vi "ds get index by serial number.vi"(10 "docking_station_index":u32, 11 "serial_number":u32) -> (2 "docking_station_index out":u32, 3 "function return":i32)   [LabVIEW 2019, in "apdm.lvlib"]
doc: "APDM_EXPORT int apdm_ds_get_index_by_serial_number(const uint32_t serial_number, uint32_t *docking_station_index);"
uses:
  apdm.lvlib
  Lee Lab/CP FES Walking 2018/Code/Working/LabVIEW/apdm.dll
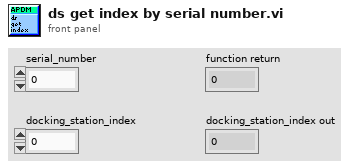
[diagram p1: front panel]
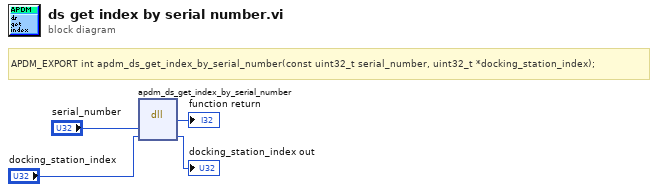
[diagram p0: block diagram]
diagram:
  # "APDM_EXPORT int apdm_ds_get_index_by_serial_number(const uint32_t serial_number, uint32_t *docking_station_index);"
  n1 = dll-call lib="C:/Users/jfalesi/Dropbox/Lee Lab/CP FES Walking 2018/Code/Working/LabVIEW/apdm.*" fn="apdm_ds_get_index_by_serial_number"("serial_number"="serial_number", "docking_station_index"="docking_station_index") -> (→"function return":i32, "docking_station_index"=→"docking_station_index out":u32)  [unwired: 4 in, 2 out]
